vi "Begin.vi"() -> (0 "error out":errorcluster)   [LabVIEW 2011]
doc: "Called before other user functions, this VI is expected to open initial I/O refnums, load in file data, and do all program initialization. Notice that the <B>error out</B> terminal is simply used for data flow. Wiring it to other structures or subVIs ensures that this VI runs first."
uses:
  <vilib>/Rock Robotics/SystemInterfaces/DIO/FPGA_DIOPWMChannel.ctl
  <vilib>/Rock Robotics/WPI/Joystick/WPI_JoystickDeviceEnum.ctl
  <vilib>/Rock Robotics/SystemInterfaces/Typedef/FPGA_TypedefSolenoidModule.ctl
  <vilib>/Rock Robotics/WPI/Solenoid/WPI_SolenoidChannel.ctl
  <vilib>/Rock Robotics/SystemInterfaces/DIO/FPGA_DIOChannel.ctl
  <vilib>/Rock Robotics/SystemInterfaces/Typedef/FPGA_TypedefDigitalModule.ctl
  <vilib>/Rock Robotics/WPI/CAN/Jaguar/SubVIs/WPI_CANJaguar_ControlMode.ctl
  <vilib>/Rock Robotics/WPI/CAN/Jaguar/SubVIs/WPI_CANJaguar_SpeedReference.ctl
  <vilib>/Rock Robotics/SystemInterfaces/DIO/FPGA_DIORelayChannel.ctl
  Robot Global Data.vi
  <vilib>/Rock Robotics/WPI/RobotDrive/WPI_RobotDriveOpen2MotorWithJaguar.vi
  <vilib>/Rock Robotics/WPI/MotorControl/WPI_MotorControlOpenCANJaguar.vi
  <vilib>/Rock Robotics/WPI/Solenoid/WPI_SolenoidOpenDouble.vi
  <vilib>/Rock Robotics/WPI/Compressor/WPI_CompressorGetSetRefNum.vi
  <vilib>/Rock Robotics/WPI/RobotDrive/WPI_RobotDriveOpen2MotorWithExistingMotors.vi
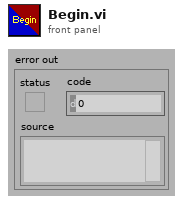
[diagram p1: front panel]
types:
  T1 = typedef "WPI_CANJaguar_ControlMode.ctl" = enum8{"Percent VBus", "Current", "Speed", "Position", "Voltage"}
  T2 = typedef "FPGA_DIORelayChannel.ctl" = enum8{"Relay 1", "Relay 2", "Relay 3", "Relay 4", "Relay 5", "Relay 6", "Relay 7", "Relay 8", "Invalid"}
  T3 = typedef "FPGA_DIOChannel.ctl" = enum8{"DIO 1", "DIO 2", "DIO 3", "DIO 4", "DIO 5", "DIO 6", "DIO 7", "DIO 8", "DIO 9", "DIO 10", "DIO 11", "DIO 12", "DIO 13", "DIO 14", "Invalid"}
  T4 = typedef "FPGA_TypedefDigitalModule.ctl" = enum16{"Digital Module 1", "Digital Module 2"}
  T5 = typedef "WPI_CANJaguar_SpeedReference.ctl" = u8
  T6 = typedef "WPI_SolenoidChannel.ctl" = enum8{"Solenoid 1", "Solenoid 2", "Solenoid 3", "Solenoid 4", "Solenoid 5", "Solenoid 6", "Solenoid 7", "Solenoid 8", "Invalid"}
  T7 = typedef "FPGA_TypedefSolenoidModule.ctl" = enum16{"Solenoid Module 1", "Solenoid Module 2"}
  T8 = typedef "WPI_JoystickDeviceEnum.ctl" = enum16{"USB 1", "USB 2", "USB 3", "USB 4", "Kinect 1", "Kinect 2"}
  T9 = typedef "FPGA_DIOPWMChannel.ctl" = enum8{"PWM 1", "PWM 2", "PWM 3", "PWM 4", "PWM 5", "PWM 6", "PWM 7", "PWM 8", "PWM 9", "PWM 10", "Invalid"}
  T10 = typedef "WPI_MotorControlDeviceRef.ctl" = cluster{"DeviceStatus":errorcluster, "Type":enum16{"PWM", "CAN"}, "PWM":cluster{"Digital Module":T4, "PWM Channel":T9, "DeadBand":T11}, "CAN":cluster{"Device Number":u8, "Control Mode":T1, "Semaphore":T12, "Max Vout":dbl}, "Invert":bool, "TransformRef":T13, "InvTransformRef":T13}
  T11 = typedef "WPI_PWMDeadband.ctl" = cluster{"Name":string, "maxPositivePwm":i32, "minPositivePwm":i32, "centerPwm":i32, "maxNegativePwm":i32, "minNegativePwm":i32, "angularRange":u16}
  T12 = typedef "Semaphore RefNum" = refnum<k1>
  T13 = typedef "WPI_PWMTransform_ConPane.ctl" = refnum<vi>
  T14 = typedef "WPI_RobotDriveDevRef.ctl" = cluster{"DevStatus":errorcluster, "Motors[]":T10[], "Square Inputs":bool, "Max Output":dbl, "Isochronous":bool}
  T15 = typedef "WPI_JoystickDevRef.ctl" = cluster{"Device":T8}
  T16 = typedef "WPI_DigitalInputDevRef.ctl" = cluster{"DevStatus":errorcluster, "DIO Channel":T3, "Digital Module":T4}
  T17 = typedef "WPI_DigitalOutputDevRef.ctl" = cluster{"Digital Module":T4, "DIO Channel":T3, "DevStatus":errorcluster}
  T18 = typedef "WPI_CompressorDevRef.ctl" = cluster{"DevStatus":errorcluster, "DigitalInputDevRef":T16, "RelayDevRef":T19}
  T19 = typedef "WPI_RelayDevRef.ctl" = cluster{"DevStatus":errorcluster, "Relay Channel":T2, "Digital Module":T4, "Relay Direction":T20}
  T20 = typedef "WPI_RelayDirection.ctl" = enum16{"Both directions", "Forward only", "Reverse only"}
  T21 = typedef "WPI_SolenoidDevRef.ctl" = cluster{"DevStatus":errorcluster, "Solenoid Module":T7, "Forward Solenoid Channel":T6, "Reverse Solenoid Channel":T6}
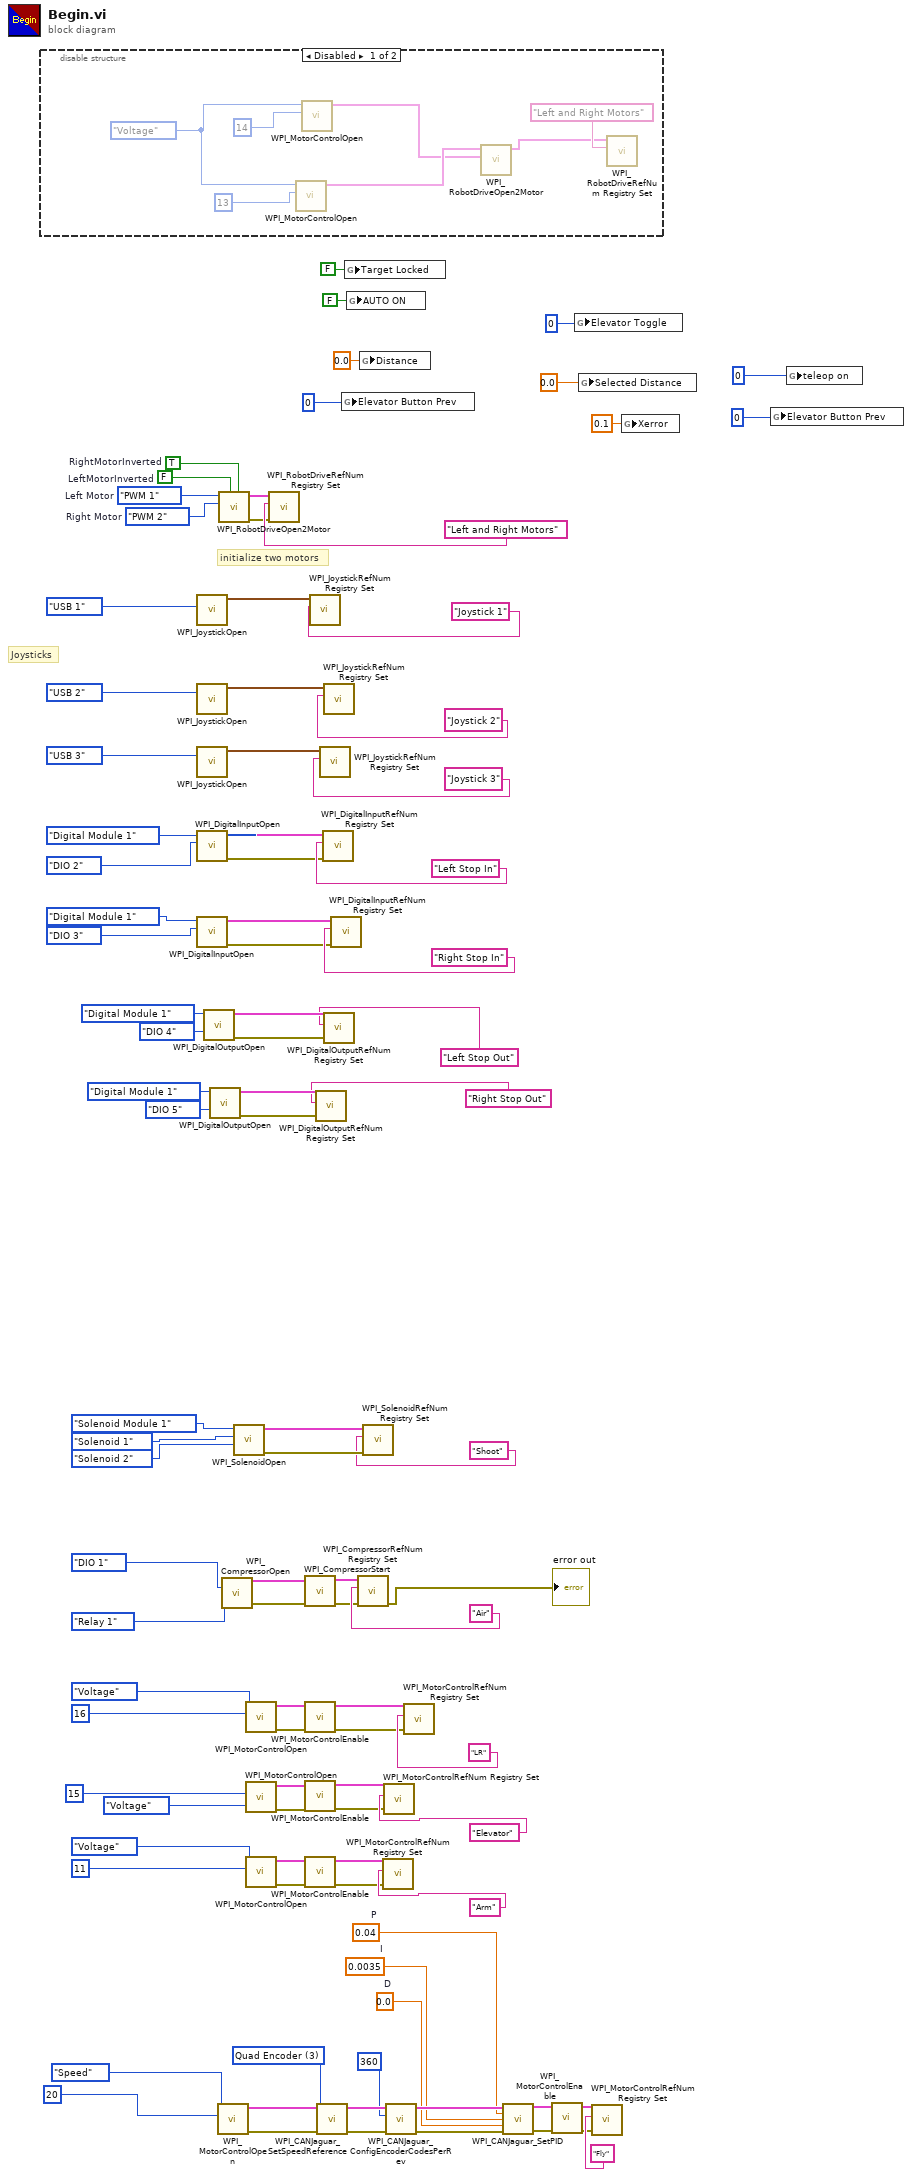
[diagram p0: block diagram]
diagram:
  w37 = 0.0  # D
  w38 = 0.0035  # I
  w39 = 0.04  # P
  w43 = T5 3 items=["Encoder"=0, "Inv Encoder"=2, "Quad Encoder"=3, "None"=255] ("Speed Reference")
  w91 = FPGA_DIOPWMChannel."PWM 2"  # Right Motor
  w92 = FPGA_DIOPWMChannel."PWM 1"  # Left Motor
  w96 = FALSE  # LeftMotorInverted
  w97 = TRUE  # RightMotorInverted
  # "Joysticks"
  # "initialize two motors"
  n1 = disable-structure shown="Disabled" {
    frame Disabled {
      w105 = WPI_CANJaguar_ControlMode."Voltage" ("Control Mode")
      n2 = call-poly <vilib>:"WPI_MotorControlOpen.vi"("Device Number"=u8 13, "Control Mode"=w105) -> ("MotorControlDeviceRef"=w100:T10)  [unwired: 8 in, 1 out]
      n3 = call-poly <vilib>:"WPI_MotorControlOpen.vi"("Device Number"=u8 14, "Control Mode"=w105) -> ("MotorControlDeviceRef"=w99:T10)  [unwired: 8 in, 1 out]
      n4 = call-poly <vilib>:"WPI_RobotDriveOpen2Motor.vi"("Right Motor Dev Ref"=w99, "Left Motor Dev Ref"=w100) -> ("RobotDriveDevRef"=w101:T14)  [unwired: 8 in, 1 out]
      n5 = call <vilib>:"WPI_RobotDriveRefNum Registry Set.vi"("refnum name"="Left and Right Motors", "RobotDriveDevRef"=w101) -> ()  [unwired: 1 in, 9 out]
    }
    frame Enabled {
    }
  }
  n6 = call <vilib>:"WPI_JoystickOpen.vi"("JoystickDevice"=WPI_JoystickDeviceEnum."USB 1") -> ("JoystickDevRef"=w84:T15)  [unwired: 10 out]
  n7 = call <vilib>:"WPI_JoystickOpen.vi"("JoystickDevice"=WPI_JoystickDeviceEnum."USB 2") -> ("JoystickDevRef"=w80:T15)  [unwired: 10 in]
  n8 = call <vilib>:"WPI_JoystickOpen.vi"("JoystickDevice"=WPI_JoystickDeviceEnum."USB 3") -> ("JoystickDevRef"=w77:T15)  [unwired: 10 in]
  n9 = call <vilib>:"WPI_DigitalInputOpen.vi"("DIO Channel"=FPGA_DIOChannel."DIO 2", "Digital Module (Module 1)"=FPGA_TypedefDigitalModule."Digital Module 1") -> ("error out"=w48:errorcluster, "DigitalInputDevRef"=w61:T16)  [unwired: 8 in]
  n10 = call <vilib>:"WPI_DigitalInputOpen.vi"("DIO Channel"=FPGA_DIOChannel."DIO 3", "Digital Module (Module 1)"=FPGA_TypedefDigitalModule."Digital Module 1") -> ("error out"=w51:errorcluster, "DigitalInputDevRef"=w57:T16)  [unwired: 8 in]
  n11 = call <vilib>:"WPI_DigitalOutputOpen.vi"("DIO Channel"=FPGA_DIOChannel."DIO 4", "Digital Module (Module 1)"=FPGA_TypedefDigitalModule."Digital Module 1") -> ("error out"=w29:errorcluster, "DigitalOutputDevRef"=w30:T17)  [unwired: 8 in]
  n12 = call <vilib>:"WPI_DigitalOutputOpen.vi"("DIO Channel"=FPGA_DIOChannel."DIO 5", "Digital Module (Module 1)"=FPGA_TypedefDigitalModule."Digital Module 1") -> ("error out"=w27:errorcluster, "DigitalOutputDevRef"=w26:T17)  [unwired: 8 in]
  n13 = call-poly <vilib>:"WPI_MotorControlOpen.vi"("Device Number"=u8 20, "Control Mode"=WPI_CANJaguar_ControlMode."Speed") -> ("error out"=w47:errorcluster, "MotorControlDeviceRef"=w46:T10)  [unwired: 8 in]
  n14 = call-poly <vilib>:"WPI_RobotDriveOpen2Motor.vi"("Right Motor Inverted"=w97, "Left Motor Inverted"=w96, "Right Motor"=w91, "Left Motor"=w92) -> ("error out"=w93:errorcluster, "RobotDriveDevRef"=w95:T14)  [unwired: 1 in, 5 out]
  n15 = call <vilib>:"WPI_CompressorOpen.vi"("Pressure Switch DIO Channel"=FPGA_DIOChannel."DIO 1", "Relay Channel"=FPGA_DIORelayChannel."Relay 1") -> ("CompressorDevRef"=w21:T18, "error out"=w20:errorcluster)  [unwired: 12 in]
  n16 = call-poly <vilib>:"WPI_SolenoidOpen.vi"("Reverse Solenoid Channel"=WPI_SolenoidChannel."Solenoid 2", "Forward Solenoid Channel"=WPI_SolenoidChannel."Solenoid 1" ("Solenoid Channel"), "Solenoid Module (Module 1)"=FPGA_TypedefSolenoidModule."Solenoid Module 1") -> ("error out"=w73:errorcluster, "SolenoidDevRef"=w72:T21)  [unwired: 7 in]
  n17 = call-poly <vilib>:"WPI_MotorControlOpen.vi"("Device Number"=u8 16, "Control Mode"=WPI_CANJaguar_ControlMode."Voltage") -> ("error out"=w68:errorcluster, "MotorControlDeviceRef"=w67:T10)  [unwired: 8 in]
  n18 = call-poly <vilib>:"WPI_MotorControlOpen.vi"("Device Number"=u8 15, "Control Mode"=WPI_CANJaguar_ControlMode."Voltage") -> ("error out"=w9:errorcluster, "MotorControlDeviceRef"=w8:T10)  [unwired: 8 in]
  n19 = call-poly <vilib>:"WPI_MotorControlOpen.vi"("Device Number"=u8 11, "Control Mode"=WPI_CANJaguar_ControlMode."Voltage") -> ("error out"=w14:errorcluster, "MotorControlDeviceRef"=w13:T10)  [unwired: 8 in]
  n20 = call <vilib>:"WPI_RobotDriveRefNum Registry Set.vi"("error in (no error)"=w93, "refnum name"="Left and Right Motors", "RobotDriveDevRef"=w95) -> ()  [unwired: 9 out]
  n21 = call <vilib>:"WPI_CompressorStart.vi"("error in (no error)"=w20, "CompressorDevRef"=w21) -> ("error out"=w18:errorcluster, "CompressorDevRef"=w19:T18)  [unwired: 8 in]
  n22 = call <vilib>:"WPI_MotorControlEnable.vi"("error in (no error)"=w68, "CAN Jaguar Ref"=w67) -> ("error out"=w50:errorcluster, "CAN Jaguar Ref Out"=w66:T10)  [unwired: 8 in]
  n23 = call <vilib>:"WPI_MotorControlEnable.vi"("error in (no error)"=w9, "CAN Jaguar Ref"=w8) -> ("error out"=w5:errorcluster, "CAN Jaguar Ref Out"=w7:T10)  [unwired: 8 in]
  n24 = call <vilib>:"WPI_MotorControlEnable.vi"("error in (no error)"=w14, "CAN Jaguar Ref"=w13) -> ("error out"=w4:errorcluster, "CAN Jaguar Ref Out"=w12:T10)  [unwired: 8 in]
  n25 = call <vilib>:"WPI_JoystickRefNum Registry Set.vi"("refnum name"="Joystick 1", "JoystickDevRef"=w84) -> ()  [unwired: 1 in, 9 out]
  n26 = call <vilib>:"WPI_DigitalOutputRefNum Registry Set.vi"("error in (no error)"=w27, "refnum name"="Right Stop Out", "DigitalOutputDevRef"=w26) -> ()  [unwired: 7 in, 2 out]
  n27 = call <vilib>:"WPI_CANJaguar_SetSpeedReference.vi"("error in (no error)"=w47, "Speed Reference"=w43, "CAN Jaguar Ref"=w46) -> ("error out"=w45:errorcluster, "CAN Jaguar Ref Out"=w44:T10)  [unwired: 7 in]
  n28 = call <vilib>:"WPI_JoystickRefNum Registry Set.vi"("refnum name"="Joystick 3", "JoystickDevRef"=w77) -> ()  [unwired: 8 in, 2 out]
  n29 = call <vilib>:"WPI_DigitalInputRefNum Registry Set.vi"("error in (no error)"=w48, "refnum name"="Left Stop In", "DigitalInputDevRef"=w61) -> ()  [unwired: 7 in, 2 out]
  n30 = call <vilib>:"WPI_JoystickRefNum Registry Set.vi"("refnum name"="Joystick 2", "JoystickDevRef"=w80) -> ()  [unwired: 8 in, 2 out]
  n31 = call <vilib>:"WPI_DigitalOutputRefNum Registry Set.vi"("error in (no error)"=w29, "refnum name"="Left Stop Out", "DigitalOutputDevRef"=w30) -> ()  [unwired: 7 in, 2 out]
  n32 = call <vilib>:"WPI_DigitalInputRefNum Registry Set.vi"("error in (no error)"=w51, "refnum name"="Right Stop In", "DigitalInputDevRef"=w57) -> ()  [unwired: 7 in, 2 out]
  n33 = global write "Robot Global Data.vi" "Elevator Button Prev"(u32 0 ("Camera Tilt Angle")) -> ()
  n34 = global write "Robot Global Data.vi" "Target Locked"(FALSE ("Target Locked")) -> ()
  n35 = global write "Robot Global Data.vi" "AUTO ON"(FALSE ("AUTO ON")) -> ()
  n36 = call <vilib>:"WPI_CompressorRefNum Registry Set.vi"("error in (no error)"=w18, "refnum name"="Air", "CompressorDevRef"=w19) -> ("error out"=→"error out":errorcluster)  [unwired: 7 in, 1 out]
  n37 = global write "Robot Global Data.vi" "Distance"(0.0 ("Distance")) -> ()
  n38 = call <vilib>:"WPI_SolenoidRefNum Registry Set.vi"("error in (no error)"=w73, "refnum name"="Shoot", "SolenoidDevRef"=w72) -> ()  [unwired: 7 in, 2 out]
  n39 = call <vilib>:"WPI_MotorControlRefNum Registry Set.vi"("error in (no error)"=w4, "refnum name"="Arm", "MotorControlDevRef"=w12) -> ()  [unwired: 7 in, 2 out]
  n40 = call <vilib>:"WPI_MotorControlRefNum Registry Set.vi"("error in (no error)"=w5, "refnum name"="Elevator", "MotorControlDevRef"=w7) -> ()  [unwired: 7 in, 2 out]
  n41 = call <vilib>:"WPI_CANJaguar_ConfigEncoderCodesPerRev.vi"("error in (no error)"=w45, "Encoder Codes Per Rev"=u16 360, "CAN Jaguar Ref"=w44) -> ("error out"=w40:errorcluster, "CAN Jaguar Ref Out"=w41:T10)  [unwired: 7 in]
  n42 = call <vilib>:"WPI_MotorControlRefNum Registry Set.vi"("error in (no error)"=w50, "refnum name"="LR", "MotorControlDevRef"=w66) -> ()  [unwired: 7 in, 2 out]
  n43 = call <vilib>:"WPI_CANJaguar_SetPID.vi"("CAN Jaguar Ref"=w41, "P"=w39, "I"=w38, "D"=w37, "error in (no error)"=w40) -> ("CAN Jaguar Ref Out"=w36:T10, "error out"=w35:errorcluster)  [unwired: 9 in]
  n44 = call <vilib>:"WPI_MotorControlEnable.vi"("error in (no error)"=w35, "CAN Jaguar Ref"=w36) -> ("error out"=w49:errorcluster, "CAN Jaguar Ref Out"=w53:T10)  [unwired: 8 in]
  n45 = global write "Robot Global Data.vi" "Elevator Toggle"(u32 0 ("Camera Tilt Angle")) -> ()
  n46 = global write "Robot Global Data.vi" "Selected Distance"(0.0 ("Camera Tilt Angle")) -> ()
  n47 = call <vilib>:"WPI_MotorControlRefNum Registry Set.vi"("error in (no error)"=w49, "refnum name"="Fly", "MotorControlDevRef"=w53) -> ()  [unwired: 7 in, 2 out]
  n48 = global write "Robot Global Data.vi" "Xerror"(0.1 ("Xerror")) -> ()
  n49 = global write "Robot Global Data.vi" "Elevator Button Prev"(u32 0 ("Camera Tilt Angle")) -> ()
  n50 = global write "Robot Global Data.vi" "teleop on"(u32 0 ("Camera Tilt Angle")) -> ()
